vi "Calc_Shot_Control.vi"(8 "Num Balls Stored":i16, 9 "Shot Request":bool, 10 "Shot Override":bool, 11 "Ball Shot":bool) -> (1 "Num Shots Requested":i16, 2 "Num Shots Overriden":i16, 3 "Shoot":bool)   [LabVIEW 2011]
panel:
  in  "Flywheel Up To Speed":bool
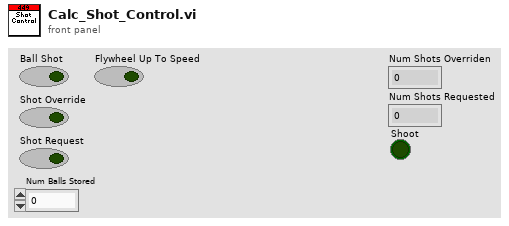
[diagram p1: front panel]
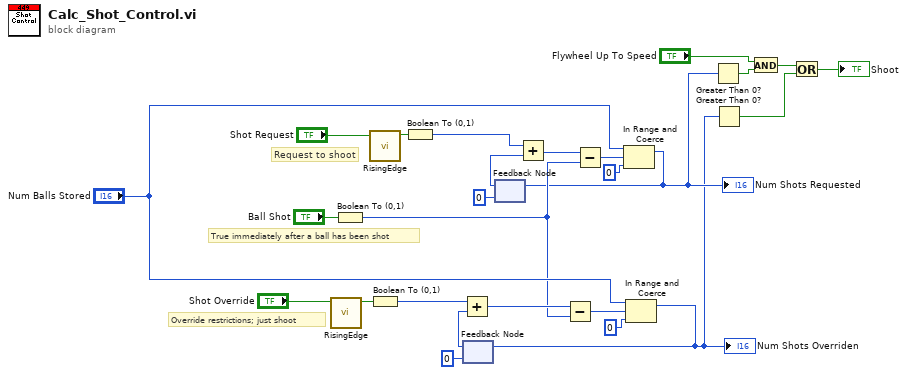
[diagram p0: block diagram]
diagram:
  # "True immediately after a ball has been shot"
  # "Request to shoot"
  # "Override restrictions; just shoot"
  n1 = call "RisingEdge.vi"("BooleanIn"="Shot Override") -> ("BooleanOut"=w24:bool)  [unwired: 10 in]
  n2 = Boolean To (0,1)(Boolean="Ball Shot") -> (0, 1=w12:i16)
  n3 = call "RisingEdge.vi"("BooleanIn"="Shot Request") -> ("BooleanOut"=w23:bool)  [unwired: 10 in]
  n4 = Boolean To (0,1)(Boolean=w24) -> (0, 1=w13:i16)
  n5 = Boolean To (0,1)(Boolean=w23) -> (0, 1=w17:i16)
  n6 = feedback #1(i16 0) -> (w22:i16)
  n7 = Add(x=w13, y=w22) -> (x+y=w20:i16)
  n8 = feedback #2(i16 0) -> (w18:i16)
  n9 = Add(x=w17, y=w18) -> (x+y=w15:i16)
  n10 = Subtract(x=w20, y=w12) -> (x-y=w9:i16)
  n11 = Subtract(x=w15, y=w12) -> (x-y=w11:i16)
  n12 = In Range and Coerce(upper limit="Num Balls Stored", x=w11, lower limit=i16 0) -> (coerced(x)=w7:i16)  [unwired: 1 out]
  "Num Shots Requested" <- w7
  n13 = feedback-in #2(w7) -> ()
  n14 = In Range and Coerce(upper limit="Num Balls Stored", x=w9, lower limit=i16 0) -> (coerced(x)=w3:i16)  [unwired: 1 out]
  "Num Shots Overriden" <- w3
  n15 = feedback-in #1(w3) -> ()
  n16 = Greater Than 0?(x=w7) -> (x > 0?=w6:bool)
  n17 = Greater Than 0?(x=w3) -> (x > 0?=w2:bool)
  n18 = And(x="Flywheel Up To Speed", y=w6) -> (x .and. y?=w4:bool)
  n19 = Or(x=w4, y=w2) -> (x .or. y?=→"Shoot":bool)
